vi "Timer.vi"(0 "Oven_Data_In":T1, 11 "Error_In":errorcluster) -> (4 "Oven_Data_Out":T1, 15 "Error_Out":errorcluster)   [LabVIEW 2023]
doc: "Used as a typical timer for the oven"
uses:
  Controls/Oven_Data.ctl
  Controls/Timer_Operation_Select.ctl
  Controls/Oven_Data_Display.ctl
  Controls/Timer_Data.ctl
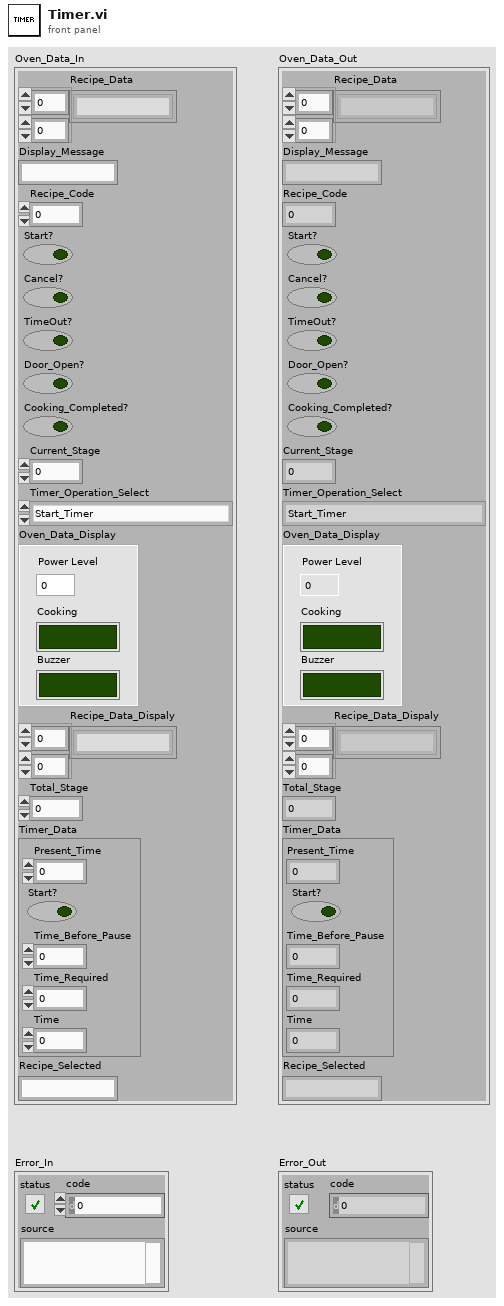
[diagram p1: front panel]
types:
  T1 = typedef "Oven_Data.ctl" = cluster{"Recipe_Data":string[][], "Display_Message":string, "Recipe_Code":i32, "Start?":bool, "Cancel?":bool, "TimeOut?":bool, "Door_Open?":bool, "Cooking_Completed?":bool, "Current_Stage":i32, "Timer_Operation_Select":T2, "Oven_Data_Display":T3, "Recipe_Data_Dispaly":string[][], "Total_Stage":i32, "Timer_Data":T4, "Recipe_Selected":string}
  T2 = typedef "Timer_Operation_Select.ctl" = enum16{"Start_Timer", "Pause_Timer", "Stop_Timer", "CheckOut_Timer"}
  T3 = typedef "Oven_Data_Display.ctl" = cluster{"Power_Level":i32, "Cooking":bool, "Buzzer":bool}
  T4 = typedef "Timer_Data.ctl" = cluster{"Present_Time":dbl, "Start?":bool, "Time_Before_Pause":dbl, "Time_Required":dbl, "Time":dbl}
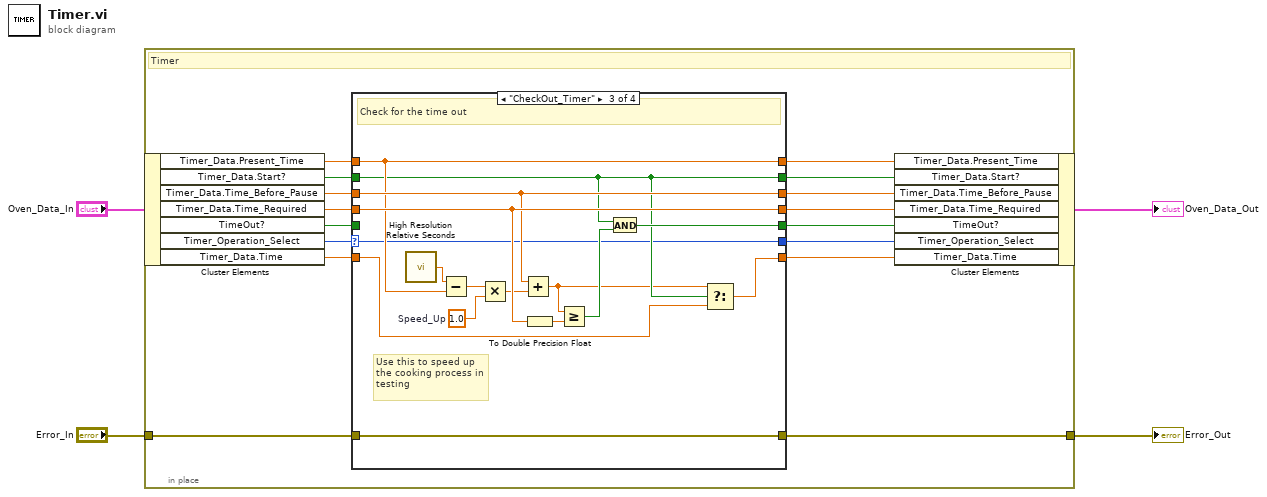
[diagram p0: block diagram]
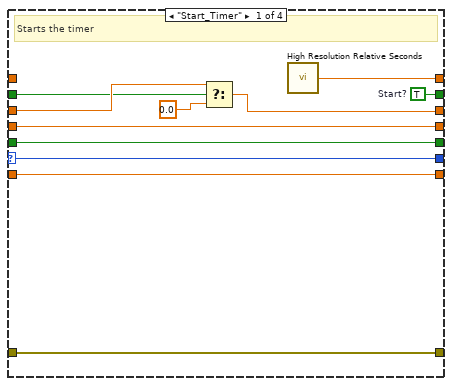
[diagram p2: hidden frame]
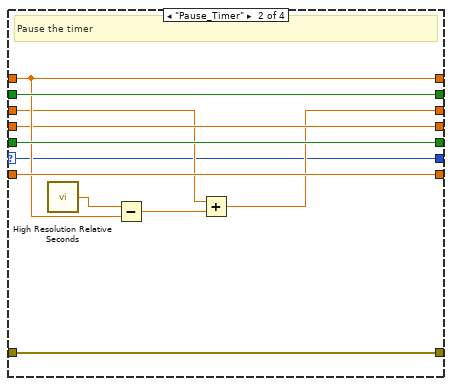
[diagram p3: hidden frame]
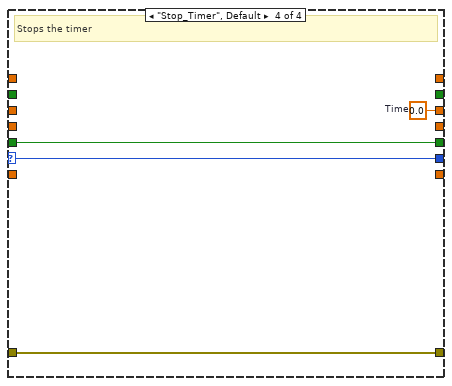
[diagram p4: hidden frame]
diagram:
  n1 = in-place {
    in-place-border: "Error_In" -> [w16]
    in-place-border: [w15] -> w3
    # "Timer"
    n2 = in-place-cluster #1("Oven_Data_In") -> ("Timer_Data.Present_Time"=w20:dbl, "Timer_Data.Start?"=w19:bool, "Timer_Data.Time_Before_Pause"=w18:dbl, "Timer_Data.Time_Required"=w17:dbl, "TimeOut?"=w7:bool, "Timer_Operation_Select"=w10:T2, "Timer_Data.Time"=w9:dbl)
    n3 = case shown="\"CheckOut_Timer\"" w10 {
      selector: w10 -> [w21 w32 w43 w59]
      tunnel: [w30 w36 w50 _] -> w12
      tunnel: w20 -> [_ w36 w50 _]
      tunnel: [w26 w40 w55 w60] -> w8
      tunnel: w16 -> [w31 w42 w57 w62]
      tunnel: [w31 w42 w57 w62] -> w15
      tunnel: [w29 w37 w49 _] -> w13
      tunnel: w19 -> [w23 w37 w49 _]
      tunnel: w17 -> [w28 w35 w54 _]
      tunnel: [w24 w33 w52 w61] -> w14
      tunnel: [w28 w35 w54 _] -> w11
      tunnel: w18 -> [w25 w34 w52 _]
      tunnel: [w27 w41 w51 _] -> w6
      tunnel: w9 -> [w27 w41 w48 _]
      tunnel: w7 -> [w26 w40 _ w60]
      tunnel: [w21 w32 w43 w59] -> w5
      frame "Start_Timer" {
        w29 = TRUE  # Start?
        # "Starts the timer"
        n4 = Select(t=w25, s=w23, f=0.0 ("t")) -> (s? t:f=w24:dbl)
        n5 = call <vilib>:"High Resolution Relative Seconds.vi"() -> ("relative seconds"=w30:dbl)
      }
      frame "Pause_Timer" {
        # "Pause the timer"
        n6 = call <vilib>:"High Resolution Relative Seconds.vi"() -> ("relative seconds"=w38:dbl)
        n7 = Subtract(x=w38, y=w36) -> (x-y=w39:dbl)
        n8 = Add(x=w34, y=w39) -> (x+y=w33:dbl)
      }
      frame "CheckOut_Timer" {
        w44 = 1.0  # Speed_Up
        # "Use this to speed up the cooking process in testing"
        # "Check for the time out"
        n9 = call <vilib>:"High Resolution Relative Seconds.vi"() -> ("relative seconds"=w56:dbl)
        n10 = Subtract(x=w56, y=w50) -> (x-y=w47:dbl)
        n11 = Multiply(x=w47, y=w44) -> (x*y=w45:dbl)
        n12 = Add(x=w52, y=w45) -> (x+y=w46:dbl)
        n13 = To Double Precision Float(number=w54) -> (double precision float=w53:dbl)
        n14 = Greater Or Equal?(x=w46, y=w53) -> (x >= y?=w58:bool)
        n15 = And(x=w49, y=w58) -> (x .and. y?=w55:bool)
        n16 = Select(t=w46, s=w49, f=w48) -> (s? t:f=w51:dbl)
      }
      frame "Stop_Timer", Default {
        w61 = 0.0  # Time
        # "Stops the timer"
      }
    }
    n17 = in-place-cluster #1("Timer_Data.Present_Time"=w12, "Timer_Data.Start?"=w13, "Timer_Data.Time_Before_Pause"=w14, "Timer_Data.Time_Required"=w11, "TimeOut?"=w8, "Timer_Operation_Select"=w5, "Timer_Data.Time"=w6) -> (→"Oven_Data_Out":T1)
  }
  "Error_Out" <- w3
